vi "Actor Core.vi"(8 "error in":errorcluster, 11 "UI Root in":refnum<class "UI Root.lvclass">) -> (0 "error out":errorcluster, 3 "Actor out":refnum<class "Actor.lvclass">)   [LabVIEW 2020, in "UI Root.lvlib" / "UI Root.lvclass"]
doc: "The user interface for this panel.\n\n----\nPlease see the following web address for additional documentation and tutorial information:\nhttp://www.mooregoodideas.com/mgi-panel-manager/\n\nAuthor: Derek Trepanier\n\nCopyright (c) 2018, Moore Good Ideas, Inc.\n\nAll rights reserved.\n\nRedistribution and use in source and binary forms, with or without modification, are permitted provided that the following conditions are met:\n\n * Redistributions of source code must retain the above copyright notice, this list of conditions and the following disclaimer.\n * Redistributions in binary form must reproduce the above copyright notice, this list of conditions and the following disclaimer in the documentation and/or other materials provided with the distribution.\n * Neither the name of Moore Good Ideas, Inc. nor the names of its contributors may be used to endorse or promote products derived from this software without specific prior written permission.\n\nTHIS SOFTWARE IS PROVIDED BY THE COPYRIGHT HOLDERS AND CONTRIBUTORS \"AS IS\" AND ANY EXPRESS OR IMPLIED WARRANTIES, INCLUDING, BUT NOT LIMITED TO, THE IMPLIED WARRANTIES OF MERCHANTABILITY AND FITNESS FOR A PARTICULAR PURPOSE ARE DISCLAIMED. IN NO EVENT SHALL THE COPYRIGHT OWNER OR CONTRIBUTORS BE LIABLE FOR ANY DIRECT, INDIRECT, INCIDENTAL, SPECIAL, EXEMPLARY, OR CONSEQUENTIAL DAMAGES (INCLUDING, BUT NOT LIMITED TO, PROCUREMENT OF SUBSTITUTE GOODS OR SERVICES; LOSS OF USE, DATA, OR PROFITS; OR BUSINESS INTERRUPTION) HOWEVER CAUSED AND ON ANY THEORY OF LIABILITY, WHETHER IN CONTRACT, STRICT LIABILITY, OR TORT (INCLUDING NEGLIGENCE OR OTHERWISE) ARISING IN ANY WAY OUT OF THE USE OF THIS SOFTWARE, EVEN IF ADVISED OF THE POSSIBILITY OF SUCH DAMAGE."
uses:
  UI Root.lvclass
  C:/Program Files/National Instruments/LabVIEW 2025/vi.lib/MGI/Panel Manager/Panel Actor/Panel Actor/Panel Actor.lvclass
  C:/Program Files/National Instruments/LabVIEW 2025/vi.lib/ActorFramework/Actor/Actor.lvclass
  <vilib>/ActorFramework/Actor/Actor.lvclass
  RFSA DAQ/RFSA DAQ/Configure VST.ctl
  UI Root.lvclass/UI Root.ctl
  <vilib>/ActorFramework/Actor/Actor.lvclass/Actor.ctl
  Application Manager/Application Manager Messages/Start TDMS Msg/Start TDMS Msg.lvclass/Start TDMS Msg.ctl
  <vilib>/ActorFramework/Message Enqueuer/Message Enqueuer.lvclass/Message Enqueuer.ctl
  Application Manager/Application Manager Messages/Start VST Msg/Start VST Msg.lvclass/Start VST Msg.ctl
  Signal Analysis/Signal Analysis/FFT Size.ctl
  Application Manager/Application Manager Messages/Set FFT Size Msg/Set FFT Size Msg.lvclass/Set FFT Size Msg.ctl
  <vilib>/ActorFramework/Message Enqueuer/Enqueue.vi
  Application Manager/Application Manager Messages/Start TDMS Msg/Start TDMS Msg.lvclass
  C:/Program Files/National Instruments/LabVIEW 2025/vi.lib/ActorFramework/Message/Message.lvclass
  Application Manager/Application Manager Messages/Start VST Msg/Start VST Msg.lvclass
  Application Manager/Application Manager Messages/Set FFT Size Msg/Set FFT Size Msg.lvclass
  Application Manager/Application Manager Messages/Stop DAQ Msg/Stop DAQ Msg.lvclass
  <vilib>/ActorFramework/Stop Msg/Stop Msg.lvclass
  <vilib>/ActorFramework/Message Priority Queue/Priority Enqueue.vi
  <vilib>/MGI/Panel Manager/Panel Actor/Panel Actor/Panel Actor.lvclass
  user32.dll
  Signal Analysis/Signal Analysis/Signal Analysis.lvclass
  RFSA DAQ/RFSA DAQ/RFSA DAQ.lvclass
panel:
  out "Title":string="G2CPU High Speed RTSA"
  in  "Window Minimize":bool
  in  "Window Maximize":bool
  in  "Close":bool
  in  "FFT Size":i32=1000000 min=32000 format="%.0p"
  in  "Run":bool
  in  "Tab Control":enum32{"TDMS", "VST"}(tab)
  in  "Threads":i32=4 min=1 max=32
  in  "Batch Size":i32=32000000 min=1 format="%#.0pS"
  in  "Source TDMS File":path
  in  "VST Config":T1={"Samples to Read per Block"=32000000, "IQ rate (S/s)"=500000000.0, "Carrier Frequency (Hz)"=1000000000.0, "Reference Level (dBm)"=0.0, "Resource Name"="RFSA", "Clock Source"="OnboardClock", "Host DMA Buffer Size"=2000000000} {"Host DMA Buffer Size" format="%.0p"; "Reference Level (dBm)" format="%.2f"; "Carrier Frequency (Hz)" format="%#.3p"; "IQ rate (S/s)" format="%#.3p"; "Samples to Read per Block" min=1 format="%.0p"}
  in  "Collapse Sidebar":bool
  in  "Stop":bool
  out "100% POI":dbl format="%#_3ps"
  out "FFT Size":dbl format="%#_3p"
  out "FFT/s":dbl format="%#_3pFFT/s"
  out "RBW:":dbl format="%#_3pHz"
  out "Throughput":dbl format="%#_3pS/s"
  out "FFT Waterfall Plot":sgl[][](graph)
  out "Signal Density Plot":sgl[][](graph)
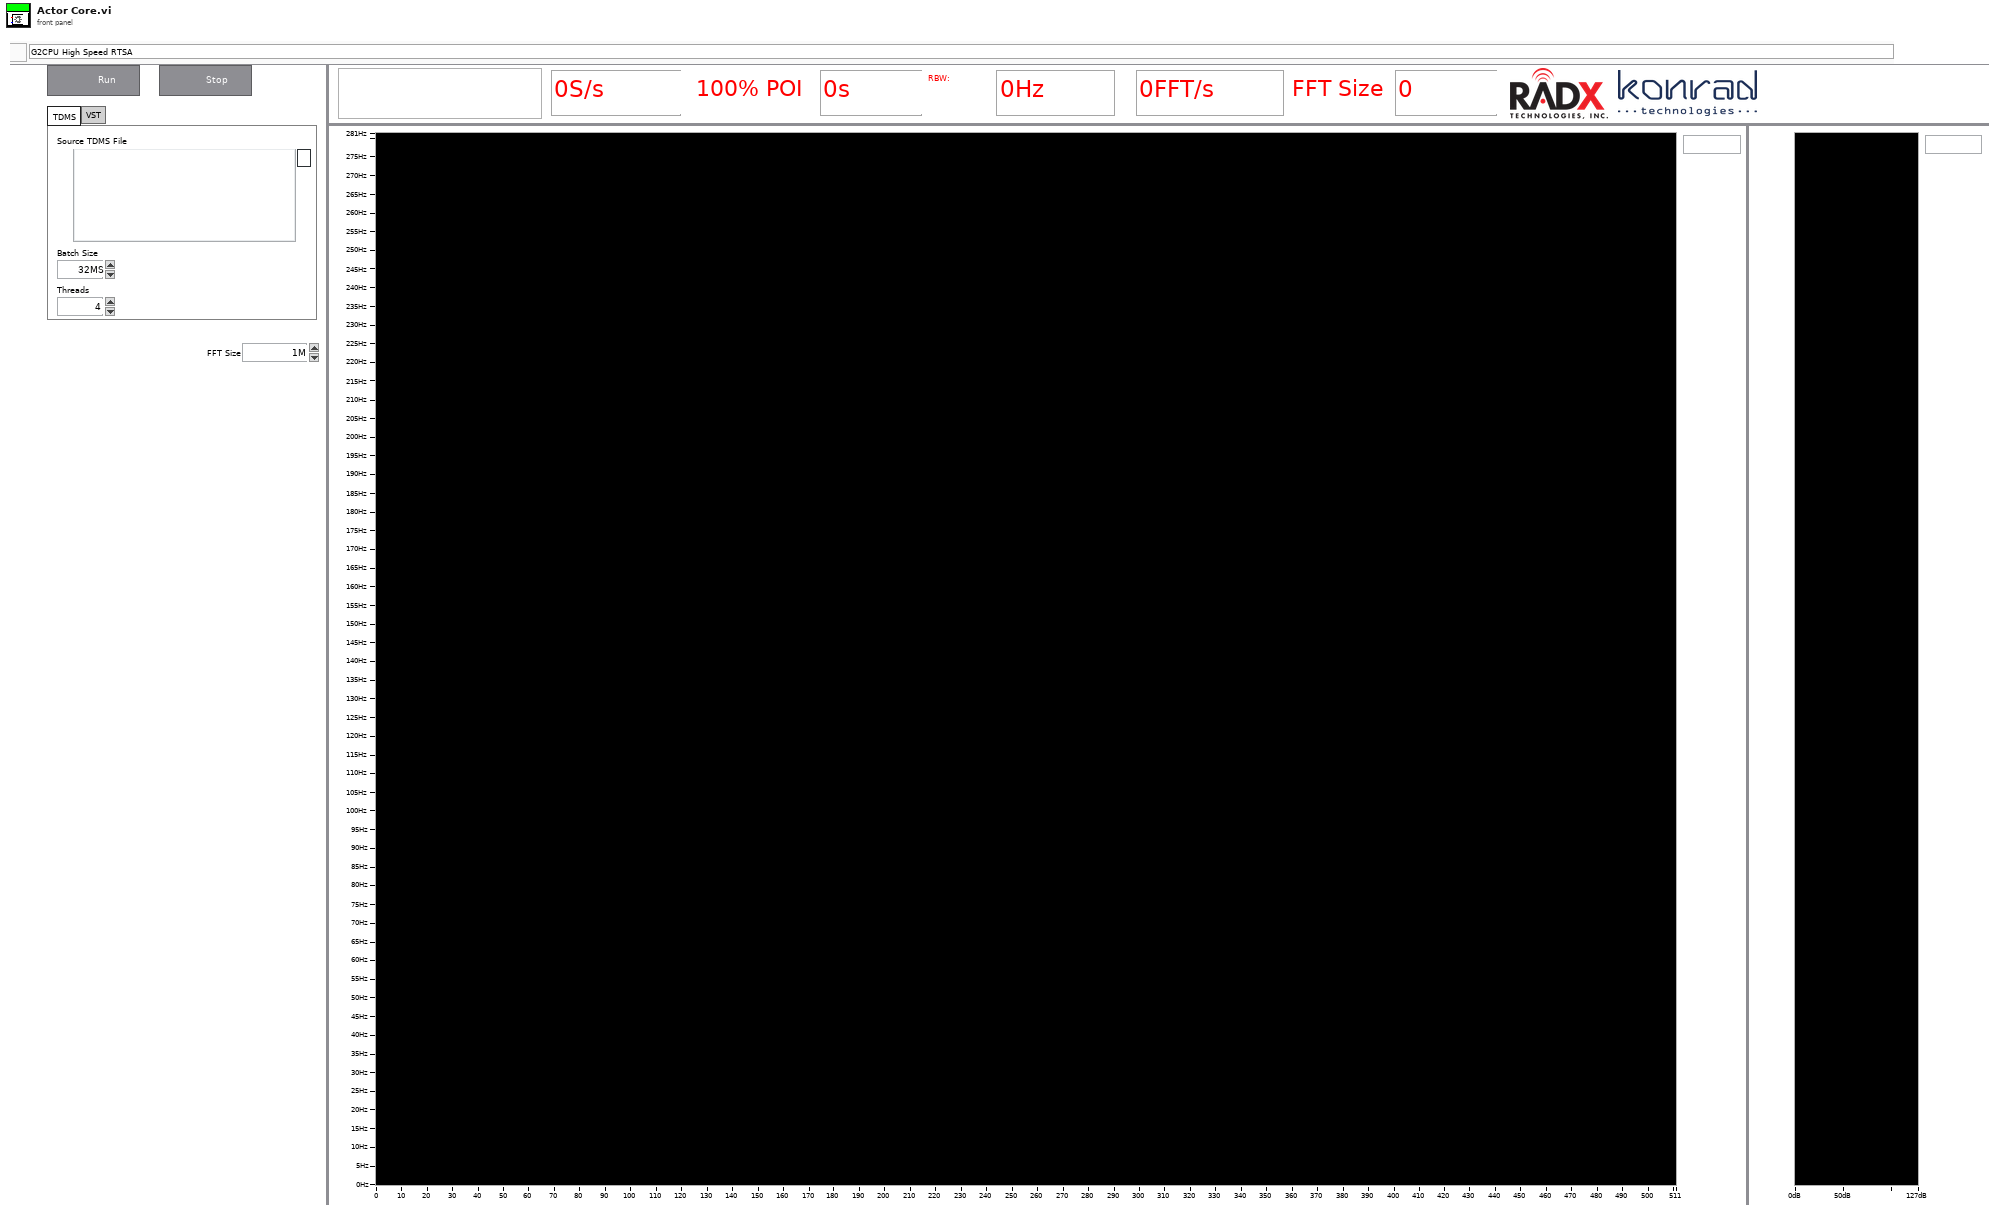
[diagram p1: front panel]
types:
  T1 = typedef "RFSA DAQ.lvlib/RFSA DAQ.lvclass/Configure VST.ctl" = cluster{"Samples to Read per Block":i32, "IQ rate (S/s)":dbl, "Carrier Frequency (Hz)":dbl, "Reference Level (dBm)":dbl, "Resource Name":refnum<k15>, "Clock Source":refnum<k15>, "Host DMA Buffer Size":i64}
  T2 = typedef "Signal Analysis.lvlib/Signal Analysis.lvclass/FFT Size.ctl" = cluster{"FFT Size":i32}
  T3 = enum32{"Invalid", "Standard", "Closed", "Hidden", "Minimized", "Maximized"}
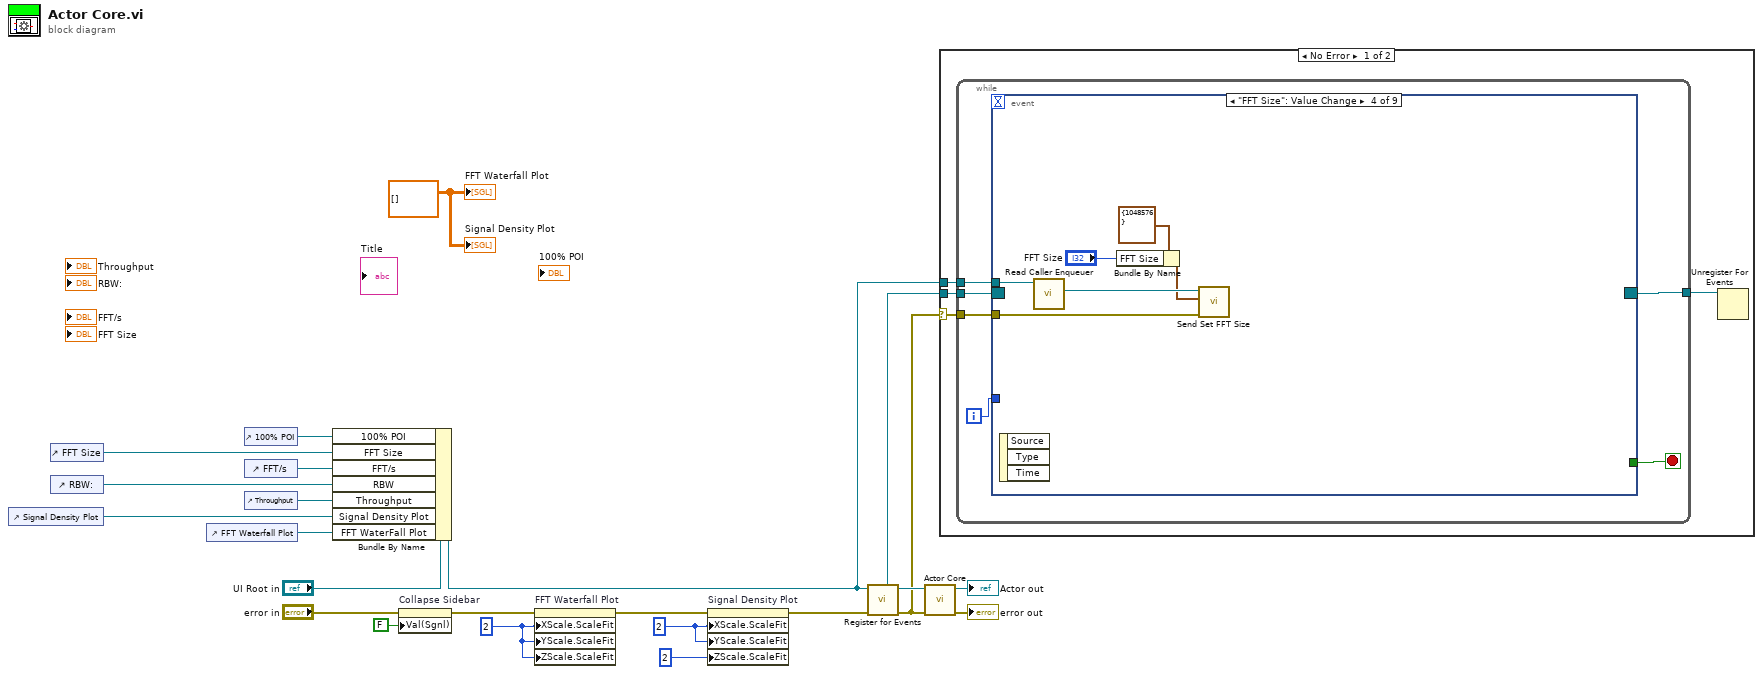
[diagram p0: block diagram]
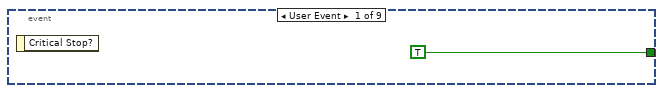
[diagram p2: hidden frame]
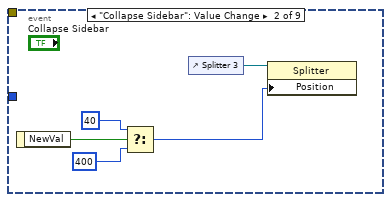
[diagram p3: hidden frame]
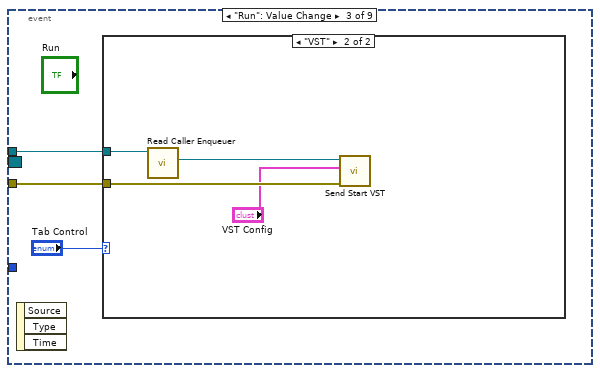
[diagram p4: hidden frame]
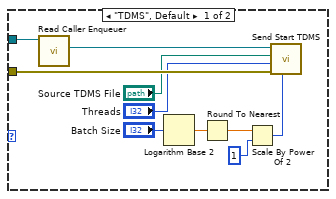
[diagram p5: hidden frame]
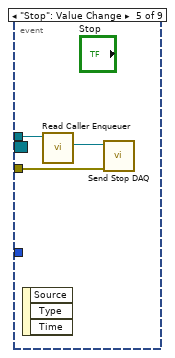
[diagram p6: hidden frame]
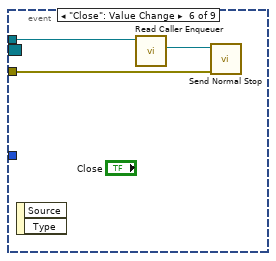
[diagram p7: hidden frame]
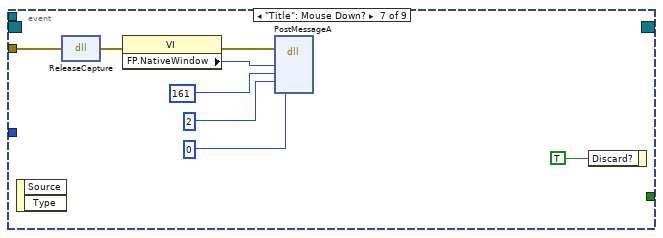
[diagram p8: hidden frame]
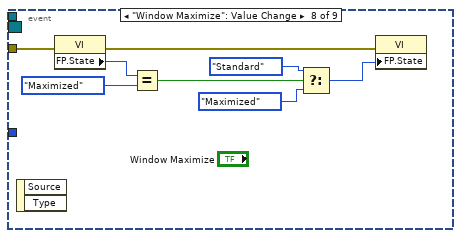
[diagram p9: hidden frame]
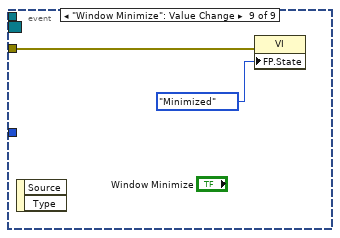
[diagram p10: hidden frame]
diagram:
  w8 = u8 2 ("X Scale.Scale Fit")
  w2 = u8 2 ("X Scale.Scale Fit")
  w12 = sgl[][] [] ("Signal Density Plot")
  n1 = control-ref of="Signal Density Plot"() -> (w11:refnum<vi>)
  n2 = control-ref of="FFT Size"() -> (w3:refnum<vi>)
  n3 = control-ref of="RBW:"() -> (w5:refnum<vi>)
  n4 = control-ref of="FFT Waterfall Plot"() -> (w13:refnum<vi>)
  n5 = control-ref of="100% POI"() -> (w1:refnum<vi>)
  n6 = control-ref of="FFT/s"() -> (w4:refnum<vi>)
  n7 = control-ref of="Throughput"() -> (w14:refnum<vi>)
  n8 = Bundle By Name(cluster="UI Root in", "100% POI"=w1, "FFT Size"=w3, "FFT/s"=w4, "RBW"=w5, "Throughput"=w14, "Signal Density Plot"=w11, "FFT WaterFall Plot"=w13) -> (w15:refnum<class "UI Root.lvclass">)
  n9 = property on="Collapse Sidebar" class="Bool (strict)"(error in="error in", "Val(Sgnl)"=FALSE ("Value (Signaling)")) -> (error out=w10:errorcluster)  [unwired: 1 in, 1 out]
  n10 = property on="FFT Waterfall Plot" class="IntChart (strict)"(error in=w10, "XScale.ScaleFit"=w2, "YScale.ScaleFit"=w2, "ZScale.ScaleFit"=w2) -> (error out=w7:errorcluster)  [unwired: 1 in, 1 out]
  n11 = property on="Signal Density Plot" class="IntGraph (strict)"(error in=w7, "XScale.ScaleFit"=w8, "YScale.ScaleFit"=w8, "ZScale.ScaleFit"=u8 2 ("Z Scale.Scale Fit")) -> (error out=w6:errorcluster)  [unwired: 1 in, 1 out]
  n12 = call <vilib>:"Register for Events.vi"("Error In"=w6, "Panel Actor in"=w15) -> ("Error Out"=w19:errorcluster, "Panel Actor out"=w21:refnum<class "UI Root.lvclass">, "Pnl Actor"=w20:refnum<event-registration>)  [unwired: 6 in, 1 out]
  n13 = call-parent "Actor Core.vi"("error in"=w19, "Panel Actor in"=w21) -> ("error out"=→"error out":errorcluster, "Actor out"=→"Actor out":refnum<class "Actor.lvclass">)  [unwired: 8 in]
  n14 = case shown="No Error" w19 {
    selector: w19 -> [w26 _]
    tunnel: w20 -> [w27 _]
    tunnel: w15 -> [w24 _]
    frame No Error {
      n15 = while {
        tunnel: w27 -> [w33]
        tunnel: w26 -> [w31]
        tunnel: [w30] -> w25
        tunnel: w24 -> [w29]
        i -> [w28]
        stop <- w32 stop-if-true
        n16 = event shown="[3] \"FFT Size\": Value Change" {
          selector: w33 -> [_ _ _ _ _ _ _ _ _]
          dyn-events: [_ _ _ _ _ _ _ _ _] -> w30
          timeout: _ -> [_ _ _ _ _ _ _ _ _]
          tunnel: [TRUE _ _ _ _ _ _ _ _] -> w32
          tunnel: w31 -> [_ _ w42 w62 w65 w66 w69 w77 w85]
          tunnel: w29 -> [_ _ w40 w60 w64 w67 _ _ _]
          tunnel: w28 -> [_ _ _ _ _ _ _ _ _]
          event User Event {
            n17 = event-data() -> ()  [unwired: 1 in, 1 out]
          }
          event "Collapse Sidebar": Value Change {
            n18 = event-data() -> ("NewVal"=w38:bool)  [unwired: 1 in]
            n19 = Select(t=40 ("Splitter Position"), s=w38, f=400) -> (s? t:f=w35:i32)
            n20 = control-ref of="Splitter 3"() -> (w39:refnum<vi>)
            n21 = property class="Splitter"(reference=w39, "Position"=w35) -> ()  [unwired: 1 in, 2 out]
          }
          event "Run": Value Change {
            n22 = event-data() -> ()  [unwired: 1 in, 3 out]
            n23 = case shown="\"VST\"" "Tab Control" {
              tunnel: w42 -> [w50 w54]
              tunnel: w40 -> [w52 w56]
              frame "TDMS", Default {
                n24 = call <vilib>:"Read Caller Enqueuer.vi"("Actor"=w52) -> ("Caller Enqueuer"=w51:refnum<class "Message Enqueuer.lvclass">)  [unwired: 10 in]
                n25 = Logarithm Base 2(1:"Batch Size") -> (0:w47:dbl)
                n26 = Round To Nearest(number=w47) -> (nearest integer value=w46:dbl)
                n27 = Scale By Power Of 2(n=w46, x=u64 1) -> (x*2^n=w43:u64)
                n28 = call "Send Start TDMS.vi"("Batch Size"=w43, "error in (no error)"=w50, "Thread Count"="Threads", "Path"="Source TDMS File", "Message Enqueuer"=w51) -> ()  [unwired: 5 in, 2 out]
              }
              frame "VST" {
                n29 = call <vilib>:"Read Caller Enqueuer.vi"("Actor"=w56) -> ("Caller Enqueuer"=w55:refnum<class "Message Enqueuer.lvclass">)  [unwired: 10 in]
                n30 = call "Send Start VST.vi"("error in (no error)"=w54, "VST Config"="VST Config", "Message Enqueuer"=w55) -> ()  [unwired: 7 in, 2 out]
              }
            }
          }
          event "FFT Size": Value Change {
            n31 = event-data() -> ()  [unwired: 1 in, 3 out]
            n32 = call <vilib>:"Read Caller Enqueuer.vi"("Actor"=w60) -> ("Caller Enqueuer"=w61:refnum<class "Message Enqueuer.lvclass">)  [unwired: 10 in]
            n33 = Bundle By Name(cluster=T2 {"FFT Size"=1048576} ("FFT Size"), "FFT Size"="FFT Size") -> (w58:T2)
            n34 = call "Send Set FFT Size.vi"("error in (no error)"=w62, "FFT Size"=w58, "Message Enqueuer"=w61) -> ()  [unwired: 7 in, 2 out]
          }
          event "Stop": Value Change {
            n35 = event-data() -> ()  [unwired: 1 in, 3 out]
            n36 = call <vilib>:"Read Caller Enqueuer.vi"("Actor"=w64) -> ("Caller Enqueuer"=w63:refnum<class "Message Enqueuer.lvclass">)  [unwired: 10 in]
            n37 = call "Send Stop DAQ.vi"("error in (no error)"=w65, "Message Enqueuer"=w63) -> ()  [unwired: 8 in, 2 out]
          }
          event "Close": Value Change {
            n38 = event-data() -> ()  [unwired: 1 in, 2 out]
            n39 = call <vilib>:"Read Caller Enqueuer.vi"("Actor"=w67) -> ("Caller Enqueuer"=w68:refnum<class "Message Enqueuer.lvclass">)  [unwired: 10 in]
            n40 = call <vilib>:"Send Normal Stop.vi"("error in (no error)"=w66, "Message Enqueuer"=w68) -> ()  [unwired: 9 in, 1 out]
          }
          event "Title": Mouse Down? {
            n41 = event-data() -> ()  [unwired: 1 in, 2 out]
            n42 = dll-call lib="user32.dll" fn="ReleaseCapture"(error in=w69) -> (error out=w75:errorcluster)  [unwired: 3 in, 1 out]
            n43 = property class="VI"(error in=w75) -> (error out=w74:errorcluster, "FP.NativeWindow"=w73:u64)  [unwired: 1 in, 1 out]
            n44 = dll-call lib="user32.dll" fn="PostMessageA"(error in=w74, "hWnd"=w73, "Msg"=161, "wParam"=2, "lParam"=0) -> ()  [unwired: 7 in, 2 out]
            n45 = event-data("Discard?"=TRUE) -> ()  [unwired: 1 in, 1 out]
          }
          event "Window Maximize": Value Change {
            n46 = event-data() -> ()  [unwired: 1 in, 2 out]
            n47 = property class="VI"(error in=w77) -> (error out=w84:errorcluster, "FP.State"=w78:T3)  [unwired: 1 in, 1 out]
            n48 = Equal?(x=w78, y=T3."Maximized" ("Front Panel Window:State")) -> (x = y?=w80:bool)
            n49 = Select(t=T3."Standard" ("Front Panel Window:State"), s=w80, f=T3."Maximized" ("Front Panel Window:State")) -> (s? t:f=w83:T3)
            n50 = property class="VI"(error in=w84, "FP.State"=w83) -> ()  [unwired: 1 in, 2 out]
          }
          event "Window Minimize": Value Change {
            n51 = event-data() -> ()  [unwired: 1 in, 2 out]
            n52 = property class="VI"(error in=w85, "FP.State"=T3."Minimized" ("Front Panel Window:State")) -> ()  [unwired: 1 in, 2 out]
          }
        }
      }
      n53 = Unregister For Events(event registration refnum=w25) -> ()  [unwired: 1 in, 1 out]
    }
    frame Error {
    }
  }
  "FFT Waterfall Plot" <- w12
  "Signal Density Plot" <- w12
